vi "Endurance.vi"(8 "error in (no error)":errorcluster, 10 "Cycles":i32=20000, 11 "instrument handle":refnum<k15>="PXI1Slot2 (62)") -> (0 "error out":errorcluster, 3 "instrument handle out":refnum<k15>="PXI1Slot2 (62)")   [LabVIEW 2018]
panel:
  out "i":i32
  out "cycle":i32
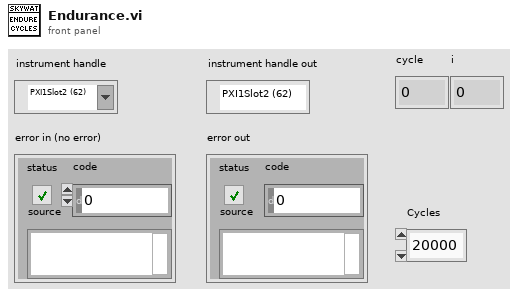
[diagram p1: front panel]
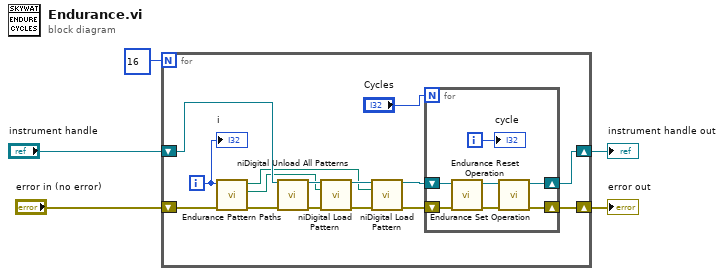
[diagram p0: block diagram]
diagram:
  n1 = for {
    N: 16 -> [_]
    shift-right: [w19] -> w4
    shift-left: "instrument handle" -> [w18]
    shift-right: [w20] -> w5
    shift-left: "error in (no error)" -> [w14]
    i -> [w15]
    n2 = call "Endurance Pattern Paths.vi"("error in (no error)"=w14, "i"=w15) -> ("error out"=w13:errorcluster, "reset path"=w8:path, "set path"=w7:path)  [unwired: 7 in]
    n3 = call <instrlib>:"niDigital Unload All Patterns.vi"("instrument handle"=w18, "error in"=w13) -> ("instrument handle out"=w16:refnum<k15>, "error out"=w17:errorcluster)  [unwired: 12 in]
    n4 = call <instrlib>:"niDigital Load Pattern.vi"("instrument handle"=w16, "pattern file"=w8, "error in"=w17) -> ("instrument handle out"=w12:refnum<k15>, "error out"=w11:errorcluster)  [unwired: 11 in]
    n5 = call <instrlib>:"niDigital Load Pattern.vi"("instrument handle"=w12, "pattern file"=w7, "error in"=w11) -> ("instrument handle out"=w10:refnum<k15>, "error out"=w9:errorcluster)  [unwired: 11 in]
    n6 = for {
      N: "Cycles" -> [_]
      shift-right: [w26] -> w19
      shift-left: w10 -> [w22]
      shift-right: [w25] -> w20
      shift-left: w9 -> [w21]
      i -> [w27]
      n7 = call "Endurance Reset Operation.vi"("error in (no error)"=w21, "instrument handle"=w22) -> ("error out"=w23:errorcluster, "instrument handle out"=w24:refnum<k15>)  [unwired: 8 in]
      n8 = call "Endurance Set Operation.vi"("error in (no error)"=w23, "instrument handle"=w24) -> ("error out"=w25:errorcluster, "instrument handle out"=w26:refnum<k15>)  [unwired: 8 in]
      "cycle" <- w27
    }
    "i" <- w15
  }
  "error out" <- w5
  "instrument handle out" <- w4
